vi "ReadConvertValiseData.vi"(4 "entrée d'erreur":errorcluster caption="entrée d'erreur (pas d'erreur)", 6 "ValiseFileIN":path, 7 "NomProjet":string) -> (0 "sortie d'erreur":errorcluster, 2 "ValiseWaveform":waveform(dbl)[](graph), 3 "ProjetOUT":string)   [LabVIEW 2017]
uses:
  <vilib>/Analysis/baseanly.llb/Mean (DBL).vi
  <vilib>/Waveform/WDTOps.llb/WDT Get Waveform Subset DBL.vi
  <vilib>/Analysis/NI_AALBase.lvlib
panel:
  out "duration":dbl
  out "AcquStartTime":timestamp
  in  "dt":dbl=0.01 format="%#_13g"
  out "last mod":timestamp
  out "VoieN":waveform(dbl)(graph)
  out "DebutVoieN":waveform(dbl)(graph)
  out "AutoZero?":bool[](array[boolean])
  out "size(s)":i32
  out "taille(s)":i32[](array[numeric])
  out "Tableau":dbl[][](array[numeric])
  out "floor(x/y)":i32
  out "taille(s) 2":i32
  out "données":waveform(dbl)[](array[waveform])
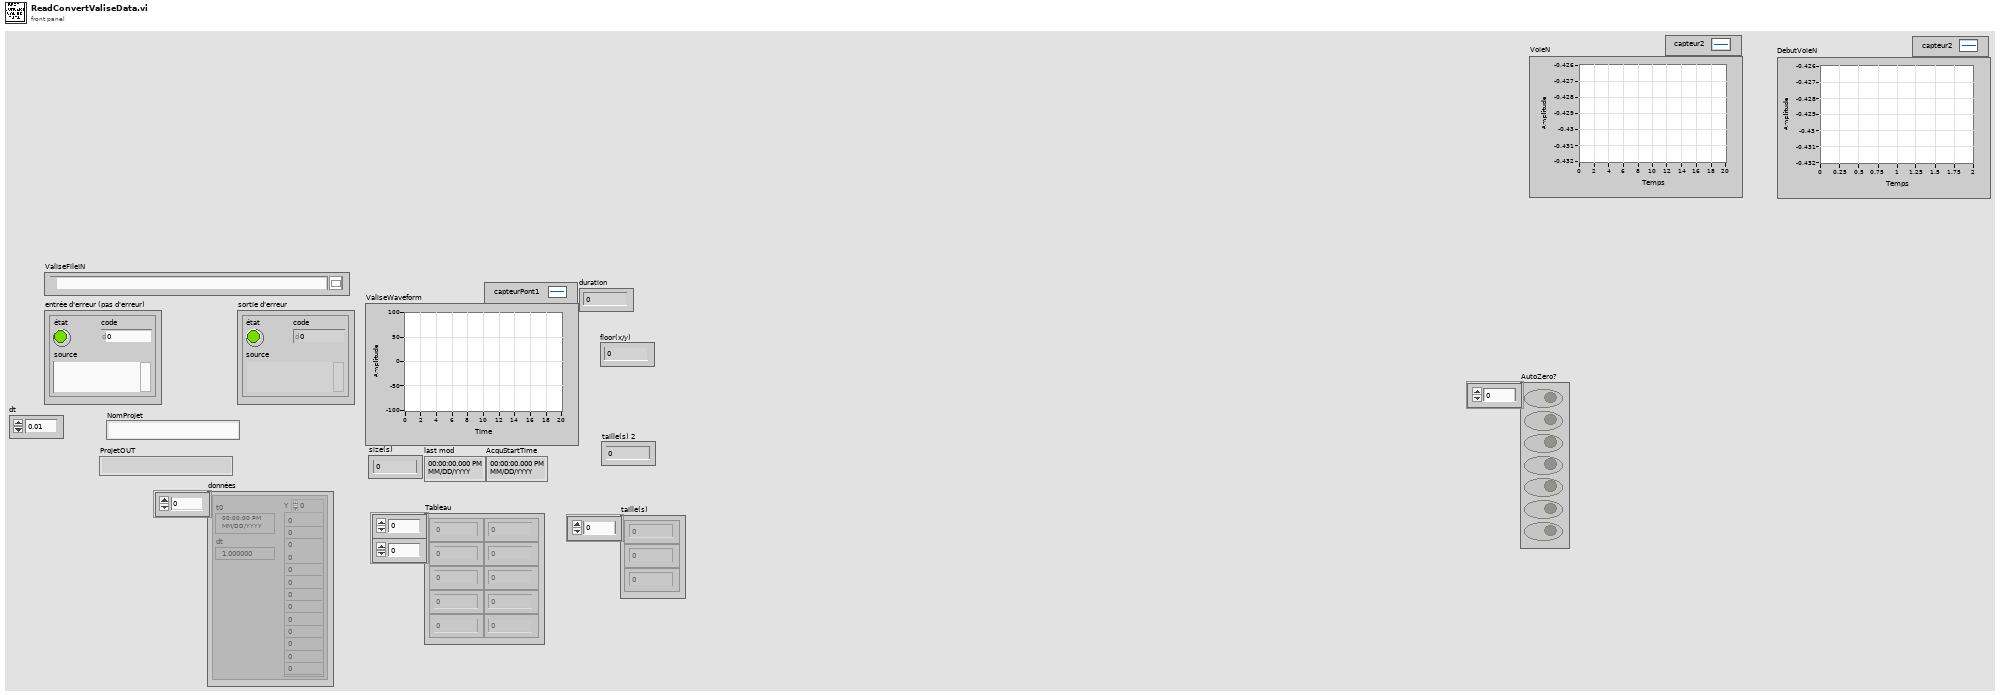
[diagram p1: front panel]
types:
  T1 = enum16{"open", "open or create", "create or replace", "create", "open (read-only)"}
  T2 = typedef "ConfigTotale.ctl" = cluster{"VoltageChannels":T3, "WheastoneBridgeChannels":T4, "Configuration":T5}
  T3 = typedef "VoltageChannels.ctl" = cluster{"ChannelNames":string[], "Sensitivity(Unit/V)":dbl[], "AutoZero":bool[], "ChannelUnits":string[], "Offsets(Units)":dbl[], "Graph Num":u8[]}
  T4 = typedef "WBridgeChannels.ctl" = cluster{"ChannelNames":string[], "Sensitivity(Unit/V)":dbl[], "AutoZero":bool[], "ChannelUnits":string[], "Offsets(Units)":dbl[], "Graph Num":u8[]}
  T5 = typedef "Configuration.ctl" = cluster{"AcqSamplingRate(Hz)":u32, "AcqTime(s)":u32, "Trigger":bool, "NbVoltageChannels":u32, "NbWBridgeChannels":u32, "Qualisys":bool, "Hexapode":bool, "FinalSamplingRate(Hz)":u32, "QualisysDataType":enum16{"6DOF", "3DTracking", "6DOF + 3D"}, "Nortek":bool, "HBM":bool}
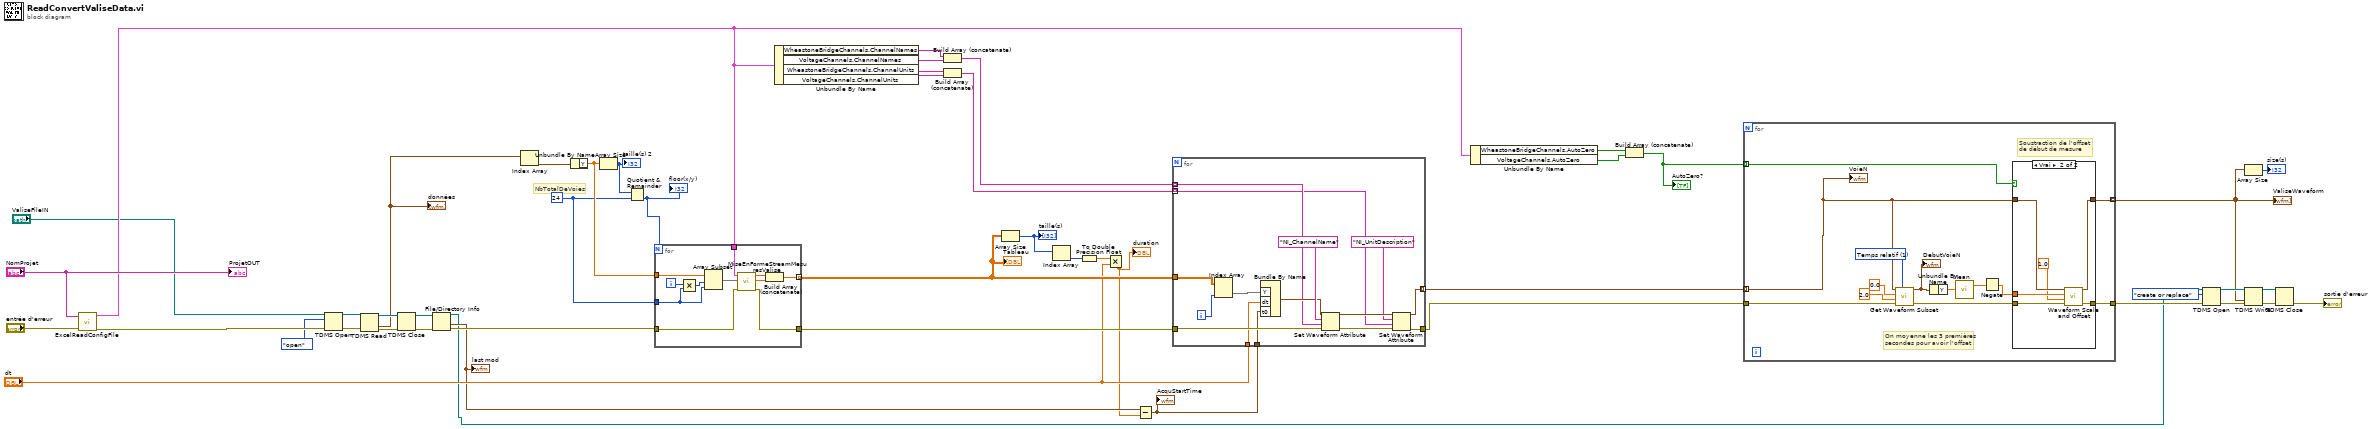
[diagram p0: block diagram]
diagram:
  w37 = 24 ("y")
  # "NbTotalDeVoies"
  n1 = call "ExcelReadConfigFile.vi"("NomProjet"="NomProjet", "error in (no error)"="entrée d'erreur") -> ("ConfigurationTotale"=w26:T2, "error out"=w12:errorcluster)  [unwired: 3 in]
  n2 = TDMS Open(8:w12, 10:T1."open" ("operation (0:open)"), 11:"ValiseFileIN") -> (0:w48:errorcluster, 3:w49:refnum<k34>)  [unwired: 4 in]
  n3 = TDMS Read(0:w49, 11:w48) -> (4:w47:refnum<k34>, 10:w38:waveform(dbl)[], 15:w46:errorcluster)  [unwired: 6 in, 3 out]
  "données" <- w38
  n4 = TDMS Close(8:w46, 11:w47) -> (0:w22:errorcluster, 3:w20:path)
  n5 = File/Directory Info(path=w20, error in=w22) -> (path out=w4:path, last mod=w15:timestamp, error out=w21:errorcluster)  [unwired: 4 out]
  "last mod" <- w15
  n6 = Index Array(array=w38) -> (element=w45:waveform(dbl))  [unwired: 1 in]
  n7 = Unbundle By Name(w45) -> ("Y"=w42:dbl[])
  n8 = Array Size(array=w42) -> (size(s)=w44:i32)
  "taille(s) 2" <- w44
  n9 = Quotient & Remainder(x=w44, y=w37) -> (floor(x/y)=w43:i32)  [unwired: 1 out]
  "floor(x/y)" <- w43
  n10 = for {
    N: w43 -> [_]
    tunnel: w42 -> [w60]
    tunnel: [w52] -> w41 mode=indexing
    tunnel: w21 -> [w56]
    tunnel: [w55] -> w40
    tunnel: w37 -> [w57]
    tunnel: w26 -> [w53]
    i -> [w59]
    n11 = Multiply(x=w59, y=w57) -> (x*y=w58:i32)
    n12 = Array Subset(array=w60, index=w58, length=w57) -> (w54:dbl[])
    n13 = call "MiseEnFormeStreamMesuresValise.vi"("Error In"=w56, "MesuresBrutesValise"=w54, "ConfigTotale"=w53) -> ("Error Out"=w55:errorcluster, "VoltageChannels1(0to15)"=w50:dbl[], "WBridgeChannels"=w51:dbl[])  [unwired: 2 in]
    n14 = Build Array (concatenate)(w51, w50) -> (w52:dbl[])
  }
  "Tableau" <- w41
  n15 = Unbundle By Name(w26) -> ("WheastoneBridgeChannels.ChannelNames"=w36:string[], "VoltageChannels.ChannelNames"=w35:string[], "WheastoneBridgeChannels.ChannelUnits"=w34:string[], "VoltageChannels.ChannelUnits"=w33:string[])
  n16 = Build Array (concatenate)(w34, w33) -> (w31:string[])
  n17 = Build Array (concatenate)(w36, w35) -> (w32:string[])
  n18 = Array Size(array=w41) -> (size(s)=w19:i32[])
  "taille(s)" <- w19
  n19 = Index Array(array=w19) -> (element=w18:i32)  [unwired: 1 in]
  n20 = To Double Precision Float(number=w18) -> (double precision float=w16:dbl)
  n21 = Multiply(x=w16, y="dt") -> (x*y=w14:dbl)
  "duration" <- w14
  n22 = Subtract(x=w15, y=w14) -> (x-y=w13:timestamp)
  "AcquStartTime" <- w13
  n23 = for {
    tunnel: w41 -> [w75]
    tunnel: [w65] -> w24 mode=indexing
    tunnel: w40 -> [w68]
    tunnel: [w67] -> w23
    tunnel: w32 -> [w64] mode=indexing
    tunnel: w31 -> [w63] mode=indexing
    tunnel: "dt" -> [w62]
    tunnel: w13 -> [w61]
    i -> [w74]
    n24 = Index Array(array=w75, index (col)=w74) -> (element=w73:dbl[])  [unwired: 1 in]
    n25 = Bundle By Name("Y"=w73, "dt"=w62, "t0"=w61) -> (w66:waveform(dbl))  [unwired: 1 in]
    n26 = Set Waveform Attribute(4:w68, 5:w64, 6:"NI_ChannelName" ("nom"), 7:w66) -> (0:w71:errorcluster, 3:w72:waveform(dbl))  [unwired: 1 out]
    n27 = Set Waveform Attribute(4:w71, 5:w63, 6:"NI_UnitDescription" ("nom"), 7:w72) -> (0:w67:errorcluster, 3:w65:waveform(dbl))  [unwired: 1 out]
  }
  n28 = Unbundle By Name(w26) -> ("WheastoneBridgeChannels.AutoZero"=w27:bool[], "VoltageChannels.AutoZero"=w28:bool[])
  n29 = Build Array (concatenate)(w27, w28) -> (w25:bool[])
  "AutoZero?" <- w25
  n30 = for {
    tunnel: w24 -> [w77] mode=indexing
    tunnel: w25 -> [w88] mode=indexing
    tunnel: w23 -> [w78]
    tunnel: [w79] -> w8
    tunnel: [w80] -> w3 mode=indexing
    w85 = u16 1 items=["Échantillons", "Temps relatif"] ("start/duration format")
    # "Soustraction de l'offset \nde début de mesure"
    # "On moyenne les 3 premières\nsecondes pour avoir l'offset"
    n31 = call-poly <vilib>:"Get Waveform Subset.vi"("start/duration format"=w85, "error in (no error)"=w78, "duration"=2.0, "start samples/time"=0.0, "waveform in"=w77) -> ("error out"=w84:errorcluster, "waveform out"=w81:waveform(dbl))  [unwired: 1 in, 2 out]
    "DebutVoieN" <- w81
    n32 = Unbundle By Name(w81) -> ("Y"=w76:dbl[])
    n33 = call-poly <vilib>:"Mean.vi"("X"=w76) -> ("mean"=w82:dbl)  [unwired: 1 out]
    n34 = Negate(x=w82) -> (-x=w83:dbl)
    n35 = case shown="Vrai" w88 {
      tunnel: w83 -> [_ w95]
      tunnel: w77 -> [w90 w96]
      tunnel: w84 -> [w89 w93]
      tunnel: [w89 w92] -> w79
      tunnel: [w90 w91] -> w80
      frame False {
      }
      frame True {
        n36 = call <vilib>:"Waveform Scale and Offset.vi"("error in (no error)"=w93, "scale"=1.0, "offset"=w95, "waveform in"=w96) -> ("error out"=w92:errorcluster, "waveform out"=w91:waveform(dbl))  [unwired: 6 in]
      }
    }
    "VoieN" <- w77
  }
  "ValiseWaveform" <- w3
  n37 = TDMS Open(8:w8, 10:T1."create or replace" ("operation (0:open)"), 11:w4) -> (0:w7:errorcluster, 3:w5:refnum<k34>)  [unwired: 4 in]
  n38 = Array Size(array=w3) -> (size(s)=→"size(s)":i32)
  n39 = TDMS Write(0:w5, 9:w3, 11:w7) -> (4:w10:refnum<k34>, 15:w9:errorcluster)  [unwired: 3 in, 2 out]
  n40 = TDMS Close(8:w9, 11:w10) -> (0:→"sortie d'erreur":errorcluster)  [unwired: 1 out]
  "ProjetOUT" <- "NomProjet"
